vi "core_rw_controls_to_file.vi"(7 "Action":T1, 8 "error in":errorcluster, 10 "ctrl refs in":refnum<vi>[](array[refnum]), 11 "config ref":T2) -> (0 "error out":errorcluster, 2 "ctrl refs out":refnum<vi>[](array[refnum]), 3 "config ref duplicate":T2)   [LabVIEW 2015]
doc: "Writes the values of an array of controls to a configuration file or reads them back.\n<b>Control References</b> is an array of the references of the controls to be saved.\n\nThe section name is the name of the VI that holds the control.\nThe key name is the label of the control."
uses:
  <vilib>/Utility/config.llb/Config Data RefNum.ctl
  Actions.ctl
  <vilib>/Utility/config.llb/Read Key (String).vi
  <vilib>/Utility/config.llb/Write Key (String).vi
  <vilib>/Utility/config.llb/NI_LVConfig.lvlib
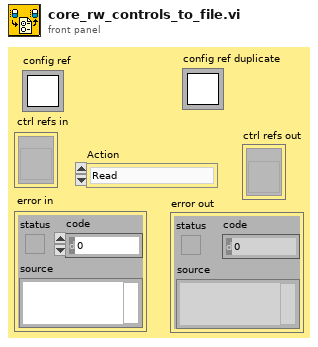
[diagram p1: front panel]
types:
  T1 = typedef "Actions.ctl" = enum16{"Read", "Write", "Read and Create"}
  T2 = typedef "NI_LVConfig.lvlib/Config Data RefNum.ctl" = refnum<k1>
  T3 = cluster{"Owning VI's name":string, "ctrl name":string, "data string":string, "Value":variant}
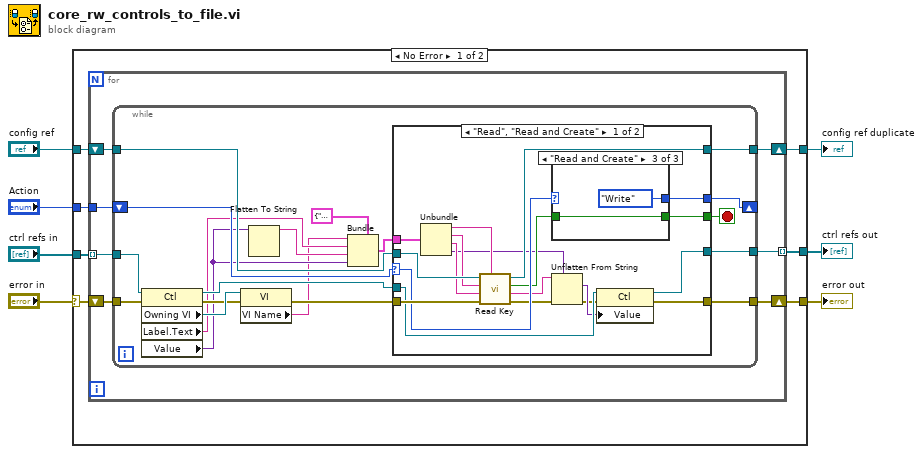
[diagram p0: block diagram]
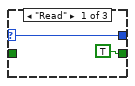
[diagram p2: hidden frame]
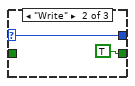
[diagram p3: hidden frame]
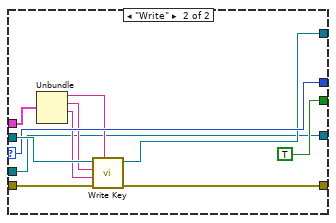
[diagram p4: hidden frame]
diagram:
  n1 = case shown="No Error" "error in" {
    selector: "error in" -> [w11 w79]
    tunnel: "ctrl refs in" -> [w14 w77]
    tunnel: [w13 w79] -> w6
    tunnel: "config ref" -> [w12 w78]
    tunnel: "Action" -> [w10 _]
    tunnel: [w9 w78] -> w3
    tunnel: [w8 w77] -> w1
    frame No Error {
      n2 = for {
        tunnel: w14 -> [w21] mode=indexing
        shift-right: [w19] -> w13
        shift-left: w11 -> [w20]
        tunnel: w10 -> [w17]
        shift-right: [w16] -> w9
        shift-left: w12 -> [w18]
        tunnel: [w15] -> w8 mode=indexing
        n3 = while {
          tunnel: w21 -> [w40]
          tunnel: w20 -> [w39]
          tunnel: [w38] -> w19
          tunnel: w18 -> [w30]
          shift-right: [w31] -> _
          shift-left: w17 -> [w32]
          tunnel: [w26] -> w16
          tunnel: [w23] -> w15
          stop <- w33 stop-if-true
          n4 = property class="Ctl"(reference=w40, error in=w39) -> (reference out=w34:refnum<vi>, error out=w36:errorcluster, "Owning VI"=w37:refnum<vi>, "Label.Text"=w29:string, "Value"=w27:variant)
          n5 = property class="VI"(reference=w37, error in=w36) -> (error out=w35:errorcluster, "VI Name"=w24:string)  [unwired: 1 out]
          n6 = Flatten To String(anything=w27) -> (data string=w28:string)  [unwired: 3 in, 2 out]
          n7 = Bundle(cluster=T3 {"Owning VI's name"="", "ctrl name"="", "data string"="", "Value"=variant}, "Owning VI's name"=w24, "ctrl name"=w29, "data string"=w28, "Value"=w27) -> (w25:T3)
          n8 = case shown="\"Read\", \"Read and Create\"" w32 {
            selector: w32 -> [w55 w72]
            tunnel: [w56 w76] -> w38
            tunnel: w30 -> [w58 w75]
            tunnel: w35 -> [w59 w74]
            tunnel: w34 -> [w57 w66]
            tunnel: [w54 TRUE] -> w33
            tunnel: [w53 w72] -> w31
            tunnel: [w47 w71] -> w26
            tunnel: w25 -> [w46 w70]
            tunnel: [w41 w66] -> w23
            frame "Read", "Read and Create" {
              n9 = Unbundle(w46) -> ("Owning VI's name"=w45:string, "ctrl name"=w44:string, "data string"=w43:string, "Value"=w42:variant)
              n10 = call-poly <vilib>:"Read Key.vi"("section"=w45, "error in (no error)"=w59, "default value"=w43, "key"=w44, "refnum"=w58) -> ("error out"=w49:errorcluster, "value"=w51:string, "found?"=w52:bool, "refnum out"=w47:T2)  [unwired: 3 in]
              n11 = case shown="\"Read and Create\"" w55 {
                selector: w55 -> [w61 w62 _]
                tunnel: [TRUE ("found?") TRUE w65] -> w54
                tunnel: [w61 w62 Actions."Write"] -> w53
                tunnel: w52 -> [_ _ w65]
                frame "Read" {
                }
                frame "Write" {
                }
                frame "Read and Create" {
                }
              }
              n12 = Unflatten From String(type=w42, binary string=w51, error in (no error)=w49) -> (value=w50:variant, error out=w48:errorcluster)  [unwired: 2 in, 1 out]
              n13 = property class="Ctl"(reference=w57, error in=w48, "Value"=w50) -> (reference out=w41:refnum<vi>, error out=w56:errorcluster)
            }
            frame "Write" {
              n14 = Unbundle(w70) -> ("Owning VI's name"=w69:string, "ctrl name"=w68:string, "data string"=w67:string)  [unwired: 1 out]
              n15 = call-poly <vilib>:"Write Key.vi"("section"=w69, "error in (no error)"=w74, "value"=w67, "key"=w68, "refnum"=w75) -> ("error out"=w76:errorcluster, "refnum out"=w71:T2)  [unwired: 4 in, 1 out]
            }
          }
        }
      }
    }
    frame Error {
    }
  }
  "error out" <- w6
  "config ref duplicate" <- w3
  "ctrl refs out" <- w1
